vi "Deney 3.3.vi"() -> ()   [LabVIEW 2018]
panel:
  out "8":bool
  out "7":bool
  out "Q3":bool
  out "Q0":bool
  out "2":bool
  out "1":bool
  out "3":bool
  out "4":bool
  out "5":bool
  out "6":bool
  out "Q2":bool
  in  "stop":bool
  out "Q1":bool
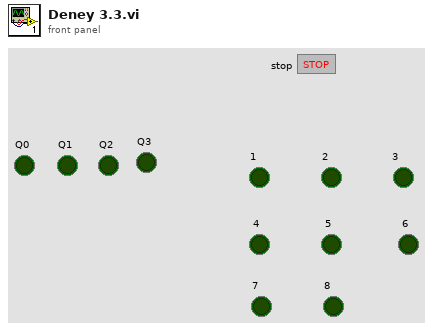
[diagram p1: front panel]
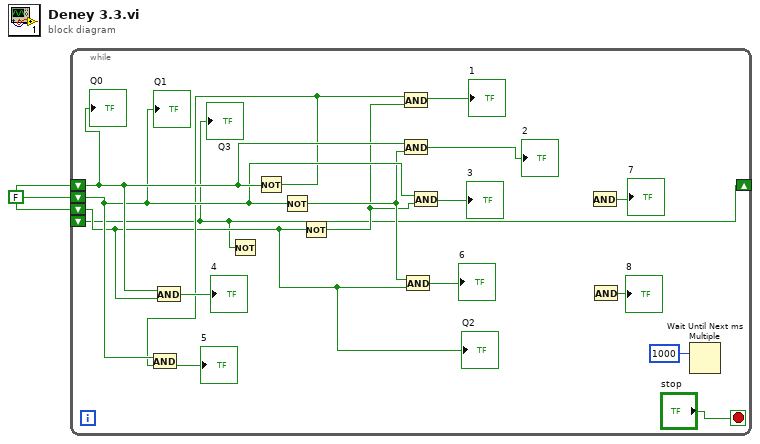
[diagram p0: block diagram]
diagram:
  w1 = FALSE
  n1 = while {
    shift-right: [w2] -> _
    shift-left: w1 -> [w13]
    shift-left: w1 -> [w12]
    shift-left: w1 -> [w6]
    shift-left: _ -> [w2]
    stop <- "stop" stop-if-true
    n2 = And(x=w13, y=w6) -> (x .and. y?=→"4":bool)
    n3 = Not(x=w2) -> ()  [unwired: 1 out]
    n4 = Not(x=w13) -> (.not. x?=w8:bool)
    n5 = And(x=w12, y=w8) -> (x .and. y?=→"5":bool)
    n6 = Not(x=w12) -> (.not. x?=w7:bool)
    n7 = Not(x=w6) -> (.not. x?=w5:bool)
    n8 = And(x=w8, y=w5) -> (x .and. y?=→"1":bool)
    n9 = And(x=w13, y=w7) -> (x .and. y?=→"2":bool)
    n10 = And(x=w7, y=w6) -> (x .and. y?=→"6":bool)
    n11 = And(x=w12, y=w5) -> (x .and. y?=→"3":bool)
    n12 = And() -> (x .and. y?=→"7":bool)  [unwired: 2 in]
    n13 = And() -> (x .and. y?=→"8":bool)  [unwired: 2 in]
    n14 = Wait Until Next ms Multiple(millisecond multiple=1000) -> ()  [unwired: 1 out]
    "Q0" <- w13
    "Q2" <- w6
    "Q1" <- w12
    "Q3" <- w2
  }
